vi "OC2 Mode.vi"(5 "coms":bool, 8 "error in (no error)":errorcluster, 10 "mode channel 1":dbl, 11 "VISA resource in":refnum<visa-resource-name>) -> (0 "error out":errorcluster, 3 "VISA resource out":refnum<visa-resource-name>)   [LabVIEW 2009]
panel:
  out "Mode string":string
  # "Mode"
  # "V1.02"
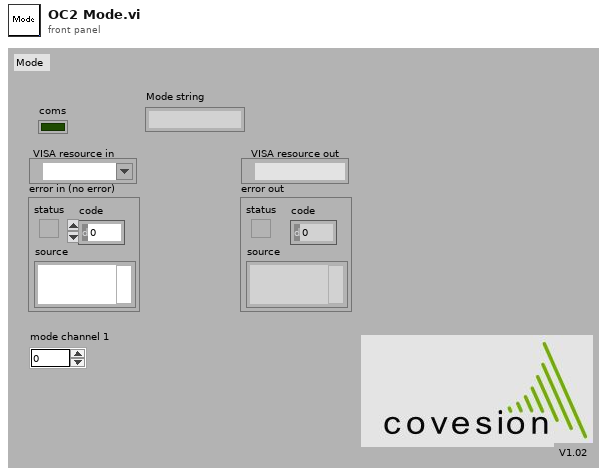
[diagram p1: front panel]
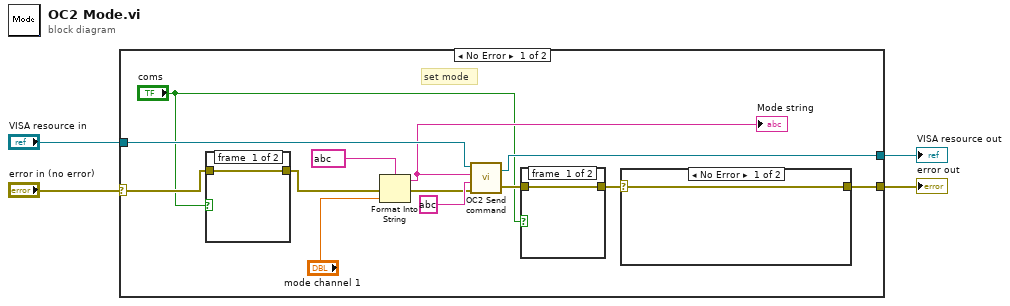
[diagram p0: block diagram]
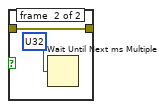
[diagram p2: hidden frame]
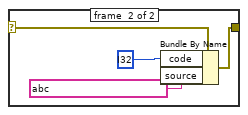
[diagram p3: hidden frame]
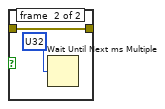
[diagram p4: hidden frame]
diagram:
  n1 = case shown="No Error" "error in (no error)" {
    selector: "error in (no error)" -> [w6 w30]
    tunnel: "VISA resource in" -> [w17 w29]
    tunnel: [w16 w29] -> w3
    tunnel: [w9 w30] -> w2
    frame #0 {
      # "set mode"
      n2 = case shown="True" "coms" {
        tunnel: [w18 w20] -> w7
        tunnel: w6 -> [w18 w20]
        frame #0 {
        }
        frame #1 {
          n3 = Wait Until Next ms Multiple(millisecond multiple=u32 ? ("milliseconds to wait")) -> ()  [unwired: 1 out]
        }
      }
      n4 = Format Into String(format string=string ?, error in=w7, "mode channel 1") -> (resulting string=w15:string, error out=w11:errorcluster)  [unwired: 1 in]
      "Mode string" <- w15
      n5 = call "OC2 Send command.vi"("VISA resource name"=w17, "Command data"=w15, "Command"=string ?, "error in (no error)"=w11) -> ("dup VISA resource name"=w16:refnum<visa-resource-name>, "error out"=w10:errorcluster)  [unwired: 1 in]
      n6 = case shown="True" "coms" {
        tunnel: [w26 w28] -> w8
        tunnel: w10 -> [w26 w28]
        frame #0 {
        }
        frame #1 {
          n7 = Wait Until Next ms Multiple(millisecond multiple=u32 ? ("milliseconds to wait")) -> ()  [unwired: 1 out]
        }
      }
      n8 = case shown="No Error" w8 {
        selector: w8 -> [w21 w25]
        tunnel: [w21 w24] -> w9
        frame #0 {
        }
        frame #1 {
          n9 = Bundle By Name(cluster=w25, "code"=i32 ?, "source"=string ?) -> (w24:errorcluster)
        }
      }
    }
    frame #1 {
    }
  }
  "error out" <- w2
  "VISA resource out" <- w3
